vi "Read Output (No Objects).vi"(8 "error in (no error)":errorcluster, 11 "Cluster In":T4={"Field"=0.0, "Rate"=0.0, "Status"={"Sweeping"=FALSE, "Clamped"=FALSE, "Hold"=FALSE, "At Rest"=FALSE, "Quench"=FALSE, "Persistent Mode"=FALSE, "Switch Heater"=FALSE}, "ILM Shut Down?"=FALSE, "IO Info"={"Address"={"Com Port"=1, "ISOBUS Address"=2, "GPIB Address"=24, "Communication"=enum."ISOBUS"}, "Version"=enum."IPS"}, "IO Info (Level Meter)"={"Address"={"Com Port"=1, "ISOBUS Address"=5, "GPIB Address"=24, "Communication"=enum."ISOBUS"}, "ILM Name"="", "Display Channel"=[]}, "Training?"=FALSE, "Training Field and Speed Cluster"={"Training Field"=[0.0, 4.108, 5.78, 8.001], "Training Speed"=[0.0057, 0.0022833333333333334, 0.0011333333333333334, 0.0011333333333333334]}}) -> (0 "error out":errorcluster, 1 "persistent?":bool, 2 "Field":dbl[unit], 3 "Cluster Out":T4={"Field"=0.0, "Rate"=0.0, "Status"={"Sweeping"=FALSE, "Clamped"=FALSE, "Hold"=FALSE, "At Rest"=FALSE, "Quench"=FALSE, "Persistent Mode"=FALSE, "Switch Heater"=FALSE}, "ILM Shut Down?"=FALSE, "IO Info"={"Address"={"Com Port"=1, "ISOBUS Address"=2, "GPIB Address"=24, "Communication"=enum."ISOBUS"}, "Version"=enum."IPS"}, "IO Info (Level Meter)"={"Address"={"Com Port"=1, "ISOBUS Address"=5, "GPIB Address"=24, "Communication"=enum."ISOBUS"}, "ILM Name"="", "Display Channel"=[]}, "Training?"=FALSE, "Training Field and Speed Cluster"={"Training Field"=[0.0, 4.108, 5.78, 8.001], "Training Speed"=[0.0057, 0.0022833333333333334, 0.0011333333333333334, 0.0011333333333333334]}}, 4 "Power supply \"field\"":dbl[unit])   [LabVIEW 2012]
uses:
  Magnet status.ctl
  Oxford/PSSUBS.LLB/PSIO.ctl
  Oxford/BUSGEN.LLB/OxfordAddress.ctl
  Power Supply.lvclass
panel:
  # "to read the output \nduring persistant mode"
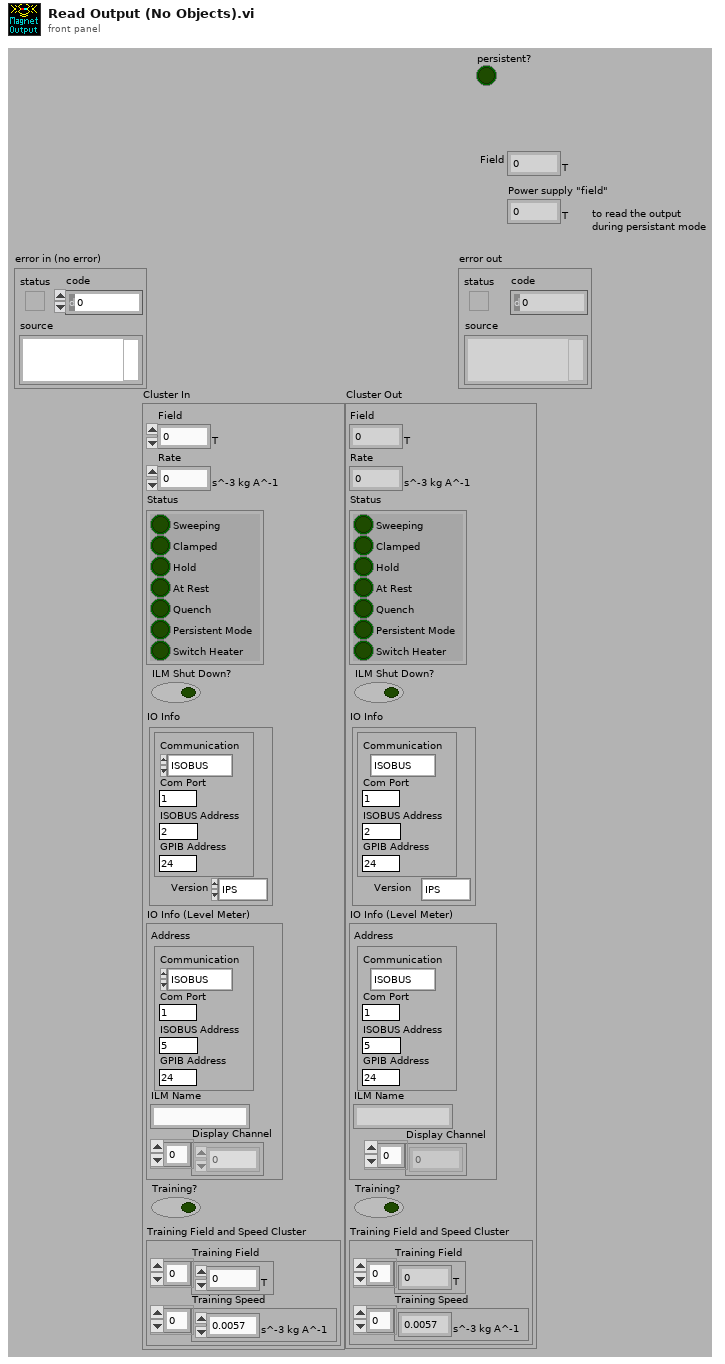
[diagram p1: front panel]
types:
  T1 = typedef "Power Supply.lvclass/Magnet status.ctl" = cluster{"Sweeping":bool, "Clamped":bool, "Hold":bool, "At Rest":bool, "Quench":bool, "Persistent Mode":bool, "Switch Heater":bool}
  T2 = typedef "PSIO.ctl" = cluster{"Address":T3, "Version":enum16{"PS", "IPS"}}
  T3 = typedef "OxfordAddress.ctl" = cluster{"Com Port":i32, "ISOBUS Address":i32, "GPIB Address":i16, "Communication":enum16{"RS232", "ISOBUS", "GPIB", "Gateway"}}
  T4 = cluster{"Field":dbl[unit], "Rate":dbl[unit], "Status":T1, "ILM Shut Down?":bool, "IO Info":T2, "IO Info (Level Meter)":cluster{"Address":T3, "ILM Name":string, "Display Channel":i32[]}, "Training?":bool, "Training Field and Speed Cluster":cluster{"Training Field":dbl[unit][], "Training Speed":dbl[unit][]}}
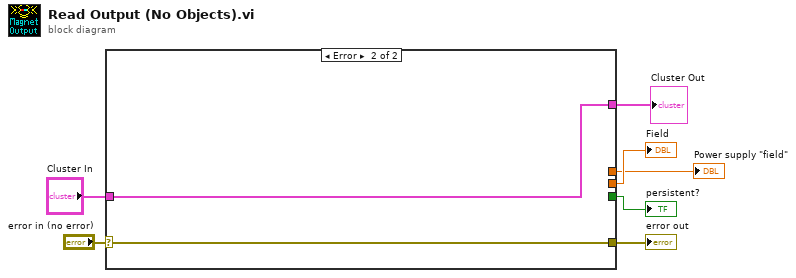
[diagram p0: block diagram]
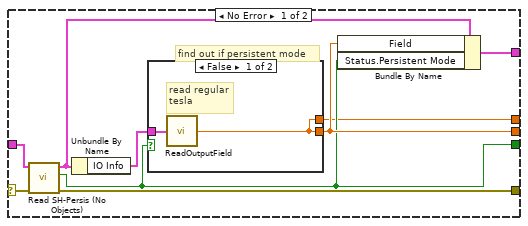
[diagram p2: hidden frame]
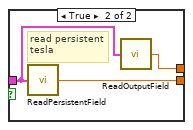
[diagram p3: hidden frame]
diagram:
  n1 = case shown="Error" "error in (no error)" {
    selector: "error in (no error)" -> [w13 w22]
    tunnel: [w10 _] -> w3
    tunnel: [w11 _] -> w2
    tunnel: "Cluster In" -> [w9 w23]
    tunnel: [w16 w22] -> w7
    tunnel: [w12 w23] -> w4
    tunnel: [w8 _] -> w1
    frame No Error {
      # "find out if persistent mode"
      n2 = call "Read SH-Persis (No Objects).vi"("error in (no error)"=w13, "Cluster In"=w9) -> ("error out"=w16:errorcluster, "pers?"=w10:bool, "Cluster Out"=w15:T4)  [unwired: 4 in, 3 out]
      n3 = Unbundle By Name(w15) -> ("IO Info"=w14:T2)
      n4 = case shown="False" w10 {
        tunnel: w14 -> [w18 w20]
        tunnel: [w17 w21] -> w11
        tunnel: [w17 w19] -> w8
        frame False {
          # "read regular\ntesla"
          n5 = call "ReadOutputField.vi"("IO Info"=w18) -> ("Field"=w17:dbl[unit])  [unwired: 2 out]
        }
        frame True {
          # "read persistent\ntesla"
          n6 = call "ReadPersistentField.vi"("IO Info"=w20) -> ("Persistent Field"=w21:dbl[unit])  [unwired: 2 out]
          n7 = call "ReadOutputField.vi"("IO Info"=w20) -> ("Field"=w19:dbl[unit])  [unwired: 2 out]
        }
      }
      n8 = Bundle By Name(cluster=w15, "Field"=w11, "Status.Persistent Mode"=w10) -> (w12:T4)
    }
    frame Error {
    }
  }
  "persistent?" <- w3
  "Field" <- w2
  "error out" <- w7
  "Cluster Out" <- w4
  "Power supply \"field\"" <- w1
